vi "Inhibit Bus A.vi"(5 "Component ID":u8, 7 "FPGA Interface":refnum<class "FPGA Interface.lvclass">, 8 "error in (no error)":errorcluster, 10 "Inhibit Bus A?":bool, 11 "1553 SubComponent in":refnum<class "1553 SubComponent.lvclass">) -> (0 "error out":errorcluster, 3 "1553 SubComponent out":refnum<class "1553 SubComponent.lvclass">)   [LabVIEW 2020, in "BCI-1553 API.lvlib" / "1553 SubComponent.lvclass"]
doc: "Inhibits or enables the operation of Bus A for the entire subcomponent."
uses:
  1553 SubComponent.lvclass
  Dependencies/FPGA Interface/FPGA Interface.lvclass
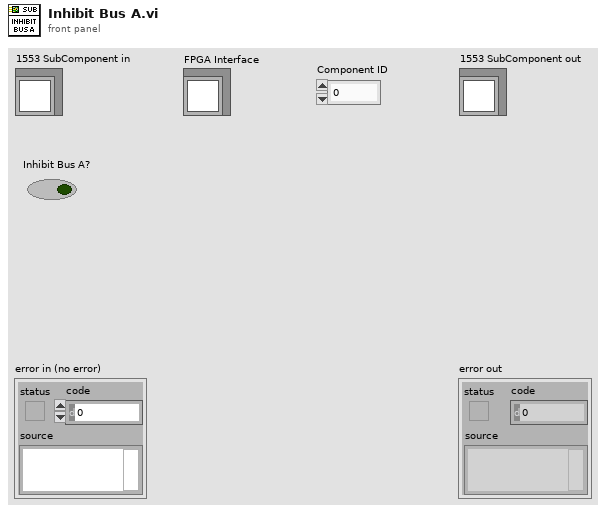
[diagram p1: front panel]
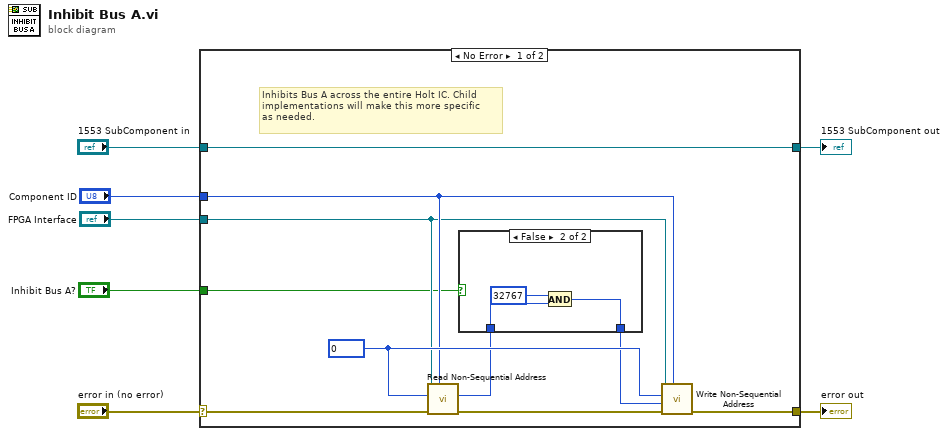
[diagram p0: block diagram]
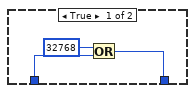
[diagram p2: hidden frame]
diagram:
  n1 = case shown="No Error" "error in (no error)" {
    selector: "error in (no error)" -> [w9 w25]
    tunnel: [w8 w25] -> w6
    tunnel: [w17 w24] -> w4
    tunnel: "1553 SubComponent in" -> [w17 w24]
    tunnel: "Component ID" -> [w12 _]
    tunnel: "FPGA Interface" -> [w11 _]
    tunnel: "Inhibit Bus A?" -> [w10 _]
    frame No Error {
      w15 = u16 0 ("Address")
      # "Inhibits Bus A across the entire Holt IC. Child\nimplementations will make this more specific\nas needed."
      n2 = call-dynamic "Read Non-Sequential Address.vi"("Target IC (1-8)"=w12, "error in (no error)"=w9, "Address"=w15, "FPGA Interface in"=w11) -> ("error out"=w16:errorcluster, "Data"=w14:u16)  [unwired: 6 in]
      n3 = case shown="False" w10 {
        tunnel: w14 -> [w20 w23]
        tunnel: [w18 w21] -> w13
        frame True {
          n4 = Or(x=u16 32768 ("Address"), y=w20) -> (x .or. y?=w18:u16)
        }
        frame False {
          n5 = And(x=u16 32767 ("Address"), y=w23) -> (x .and. y?=w21:u16)
        }
      }
      n6 = call-dynamic "Write Non-Sequential Address.vi"("Target IC (1-8)"=w12, "error in (no error)"=w16, "Data"=w13, "Address"=w15, "FPGA Interface in"=w11) -> ("error out"=w8:errorcluster)  [unwired: 6 in]
    }
    frame Error {
    }
  }
  "error out" <- w6
  "1553 SubComponent out" <- w4
